vi "UTIL_BinarySearch.vi"() -> ()   [LabVIEW 2024]
panel:
  in  "Switch":dbl
  out "PV 2":dbl
  in  "PV":dbl
  in  "B":dbl
  in  "A":dbl
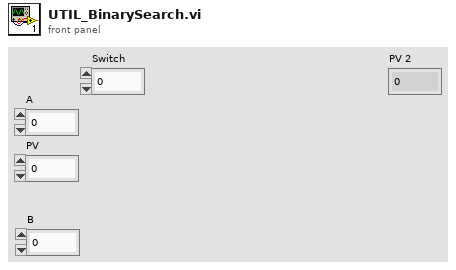
[diagram p1: front panel]
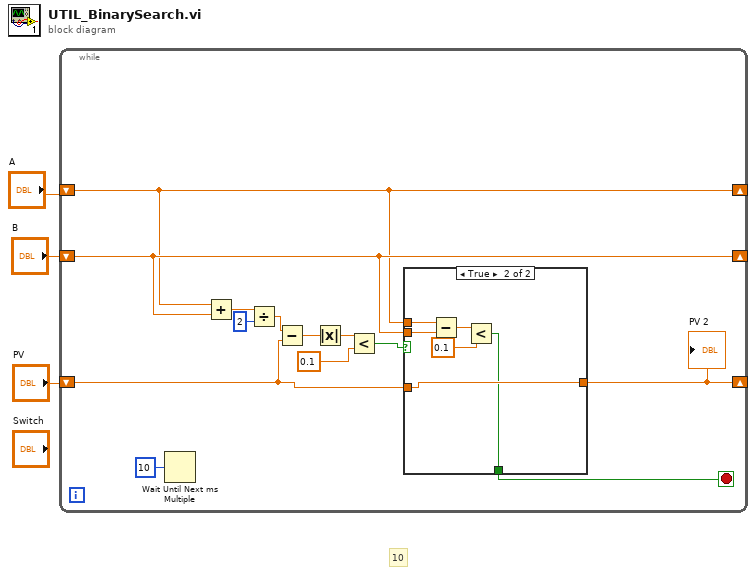
[diagram p0: block diagram]
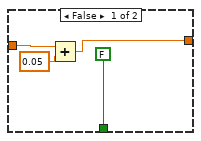
[diagram p2: hidden frame]
diagram:
  # "10"
  n1 = while {
    shift-right: [w5] -> _
    shift-left: "A" -> [w5]
    shift-right: [w6] -> _
    shift-left: "B" -> [w6]
    shift-right: [w8] -> _
    shift-left: "PV" -> [w9]
    stop <- w4 stop-if-true
    n2 = Wait Until Next ms Multiple(millisecond multiple=u32 10) -> ()  [unwired: 1 out]
    n3 = Add(x=w5, y=w6) -> (x+y=w16:dbl)
    n4 = Divide(x=w16, y=2) -> (x/y=w7:dbl)
    n5 = Subtract(x=w7, y=w9) -> (x-y=w14:dbl)
    n6 = Absolute Value(x=w14) -> (abs(x)=w13:dbl)
    n7 = Less?(x=w13, y=0.1) -> (x < y?=w10:bool)
    n8 = case shown="True" w10 {
      tunnel: w9 -> [w20 w26]
      tunnel: [w18 w26] -> w8
      tunnel: w6 -> [_ w25]
      tunnel: w5 -> [_ w24]
      tunnel: [FALSE w21] -> w4
      frame False {
        n9 = Add(x=w20, y=0.05) -> (x+y=w18:dbl)
      }
      frame True {
        n10 = Subtract(x=w24, y=w25) -> (x-y=w23:dbl)
        n11 = Less?(x=w23, y=0.1) -> (x < y?=w21:bool)
      }
    }
    "PV 2" <- w8
  }
